vi "Program_Active.vi"(0 "Hit Server Now":bool) -> ()   [LabVIEW 2017]
uses:
  ADAM Controls/Traverse_Level_State.ctl
  Anemometry/Anemometry Sub Vis/Globals/Meas_global.vi
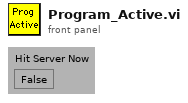
[diagram p1: front panel]
types:
  T1 = typedef "Post_Process.ctl" = enum16{"Take New Data", "Post Process Raw Data File"}
  T2 = typedef "Traverse_Level_State.ctl" = enum16{"Running", "Complete"}
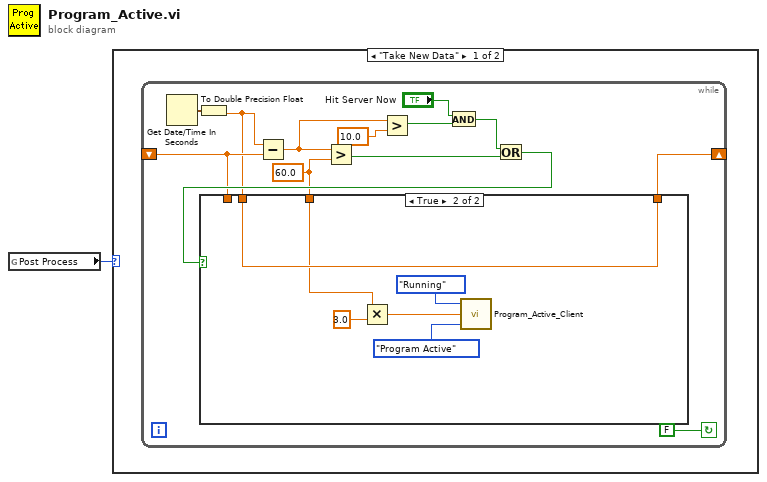
[diagram p0: block diagram]
diagram:
  n1 = global read "Meas_global.vi" "Post Process"() -> (w1:T1)
  n2 = case shown="\"Take New Data\"" w1 {
    frame "Take New Data" {
      n3 = while {
        shift-left: _ -> [w11]
        shift-right: [w12] -> _
        stop <- FALSE continue-if-true
        w2 = 60.0 ("y")
        n4 = Get Date/Time In Seconds() -> (seconds since 1Jan1904=w3:timestamp)
        n5 = To Double Precision Float(number=w3) -> (double precision float=w10:dbl)
        n6 = Subtract(x=w10, y=w11) -> (x-y=w9:dbl)
        n7 = Greater?(x=w9, y=w2) -> (0:w14:bool)
        n8 = Greater?(x=w9, y=10.0) -> (0:w6:bool)
        n9 = And(x="Hit Server Now", y=w6) -> (x .and. y?=w5:bool)
        n10 = Or(x=w5, y=w14) -> (x .or. y?=w13:bool)
        n11 = case shown="True" w13 {
          tunnel: [w15 w20] -> w12
          tunnel: w10 -> [_ w20]
          tunnel: w11 -> [w15 _]
          tunnel: w2 -> [_ w18]
          frame False {
          }
          frame True {
            n12 = Multiply(x=w18, y=3.0) -> (x*y=w16:dbl)
            n13 = call "Program_Active_Client.vi"("Mode"=enum16{"Program Active", "Traverse Level State"}."Program Active", "Time till next contact (Sec)"=w16, "Traverse level State"=Traverse_Level_State."Running") -> ()  [unwired: 3 out]
          }
        }
      }
    }
    frame "Post Process Raw Data File" {
    }
  }
